vi "TSM Relay Configuration Relay Actions to Sessions.vi"(0 "Relay Actions":T3[](array[typedef]) items=["Open Relay"=20, "Close Relay"=21], 7 "TSM Relay In":T4={"TSM context"=refnum, "Pin Query Context"=refnum, "TSM Site Numbers"=[], "SSC Relay"=[], "Unfiltered Pins"=[], "Filtered Pins"=[], "Filtered Pins Info"={"Unfiltered Pins Count"=3, "Locations"=[], "Lengths"=[]}}) -> (4 "TSM Relay Configuration Out":T1 {"SSC Relay with Action"."Relay Action" items=["Open Relay"=20, "Close Relay"=21]})   [LabVIEW 2019]
doc: "This VI maps the Relay Actions array to each SSC Relay session element, building a new array of clusters where each cluster element contains a single SSC Relay session and it's corresponding Relay Action."
uses:
  <instrlib>/niSwitch/niSwitch.llb/niSwitch Relay Action.ctl
  TSM SSC Relay.ctl
  <vilib>/NI_TestStand_SemiconductorModule/NI_TestStand_Semiconductor_Module.lvlibp/PinMap/PinQueryContext/MultiplePinMultipleSessionQueryContext/MultiplePinMultipleSessionQueryContext.lvclass
  <vilib>/NI_TestStand_SemiconductorModule/NI_TestStand_Semiconductor_Module.lvlibp/PinMap/General/SemiconductorModuleContext.ctl
  SSC/SSC Relay.ctl
  TSM Filtered Pins Info.ctl
  TSM Relay Config.ctl
  <vilib>/NI_TestStand_SemiconductorModule/NI_TestStand_Semiconductor_Module.lvlibp
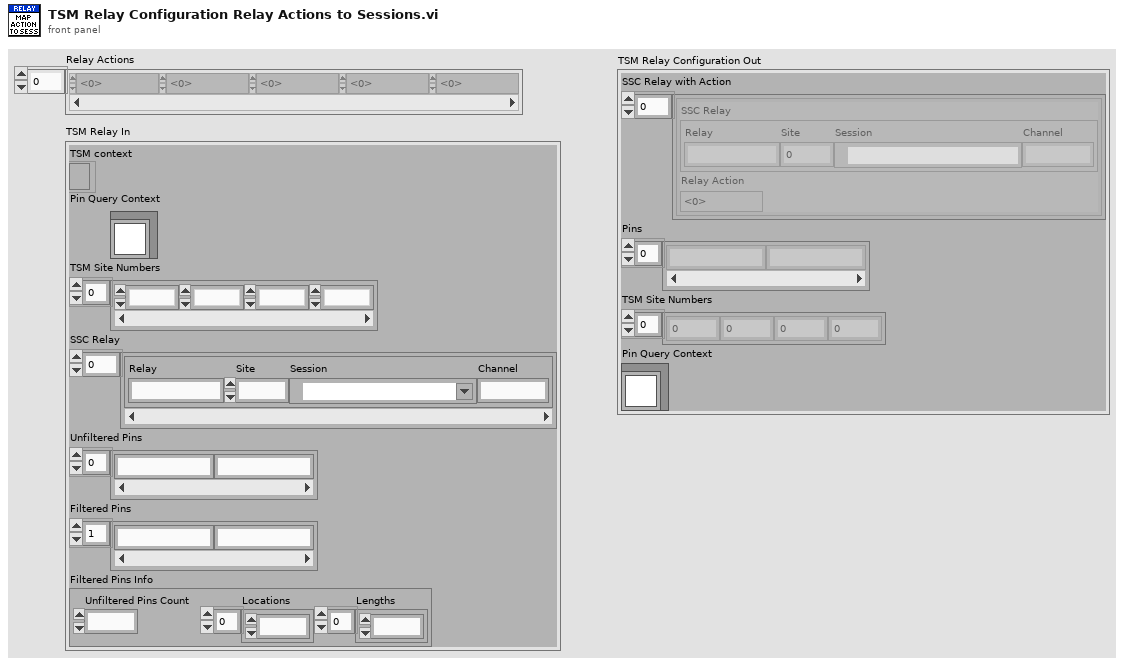
[diagram p1: front panel]
types:
  T1 = typedef "TSM Relay Config.ctl" = cluster{"SSC Relay with Action":cluster{"SSC Relay":T2, "Relay Action":T3}[], "Pins":string[], "TSM Site Numbers":i32[], "Pin Query Context":refnum<class "MultiplePinMultipleSessionQueryContext.lvclass">}
  T2 = typedef "SSC Relay.ctl" = cluster{"Relay":string, "Site":i32, "Session":refnum<k15>, "Channel":string}
  T3 = typedef "niSwitch Relay Action.ctl" = i32
  T4 = typedef "TSM SSC Relay.ctl" = cluster{"TSM context":T5, "Pin Query Context":refnum<class "MultiplePinMultipleSessionQueryContext.lvclass">, "TSM Site Numbers":i32[], "SSC Relay":T2[], "Unfiltered Pins":string[], "Filtered Pins":string[], "Filtered Pins Info":T6}
  T5 = typedef "NI_TestStand_Semiconductor_Module.lvlibp/SemiconductorModuleContext.ctl" = refnum<k7>
  T6 = typedef "TSM Filtered Pins Info.ctl" = cluster{"Unfiltered Pins Count":i32, "Locations":i32[], "Lengths":i32[]}
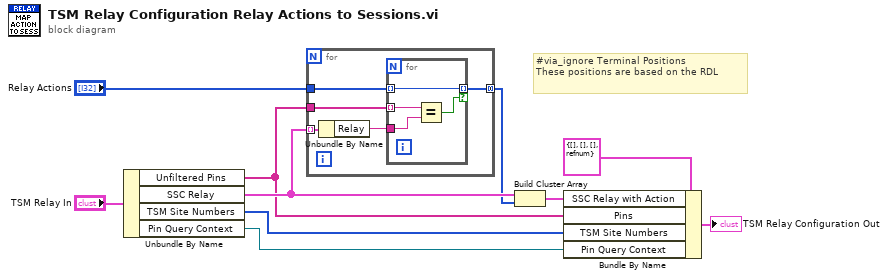
[diagram p0: block diagram]
diagram:
  # "#via_ignore Terminal Positions\nThese positions are based on the RDL"
  n1 = Unbundle By Name("TSM Relay In") -> ("Unfiltered Pins"=w2:string[], "SSC Relay"=w8:T2[], "TSM Site Numbers"=w4:i32[], "Pin Query Context"=w3:refnum<class "MultiplePinMultipleSessionQueryContext.lvclass">)
  n2 = for {
    tunnel: w2 -> [w15]
    tunnel: w8 -> [w14] mode=indexing
    tunnel: "Relay Actions" -> [w12]
    tunnel: [w11] -> w7 mode=concatenating
    n3 = Unbundle By Name(w14) -> ("Relay"=w13:string)
    n4 = for {
      tunnel: w15 -> [w19] mode=indexing
      tunnel: w13 -> [w18]
      tunnel: w12 -> [w17] mode=indexing
      tunnel: [w17] -> w11 mode=indexing if=w16
      n5 = Equal?(x=w19, y=w18) -> (x = y?=w16:bool)
    }
  }
  n6 = Build Cluster Array(w8, w7) -> (w5:cluster{"SSC":T2, "Current Level":T3}[])
  n7 = Bundle By Name(cluster=T1 {"SSC Relay with Action"=[], "Pins"=[], "TSM Site Numbers"=[], "Pin Query Context"=refnum} ("Relay Configuration"), "SSC Relay with Action"=w5, "Pins"=w2, "TSM Site Numbers"=w4, "Pin Query Context"=w3) -> (→"TSM Relay Configuration Out":T1)
